vi "Neopixel-Example Dialog.vi"(0 "Cluster In":cluster{"Numeric":dbl}, 2 "Parent VI":refnum<vi>) -> (4 "Cluster out":cluster{"Numeric":dbl}, 10 "canceled":bool)   [LabVIEW 2020]
panel:
  in  "Cancel":bool
  in  "OK":bool
  # "Put stuff here"
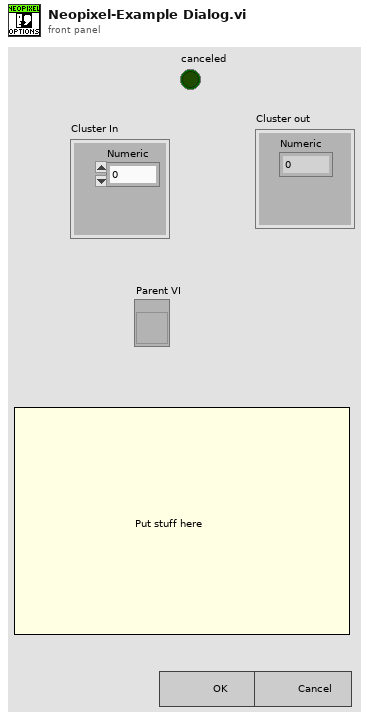
[diagram p1: front panel]
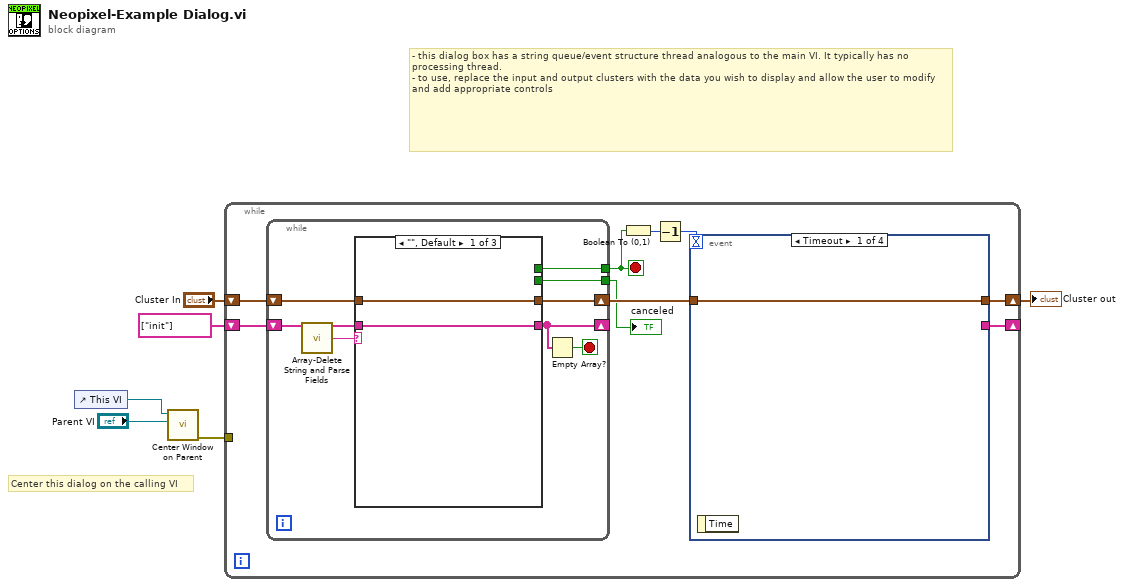
[diagram p0: block diagram]
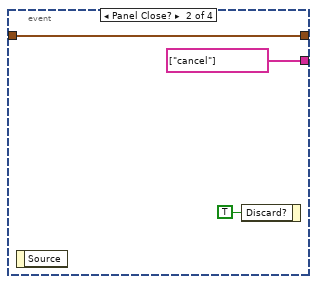
[diagram p2: hidden frame]
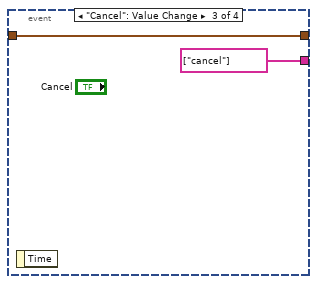
[diagram p3: hidden frame]
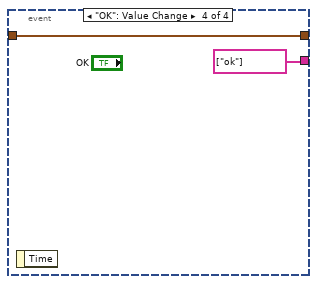
[diagram p4: hidden frame]
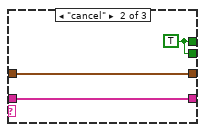
[diagram p5: hidden frame]
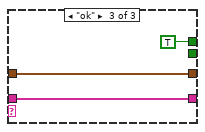
[diagram p6: hidden frame]
diagram:
  # "Center this dialog on the calling VI"
  # "- this dialog box has a string queue/event structure thread analogous to the main VI. It typically has no processing thread.\n- to use, replace the input and output clusters with the data you wish to display and allow the user to modify and add appropriate controls"
  n1 = control-ref of="This VI"() -> (w1:refnum<vi>)
  n2 = call "Center Window on Parent.vi"("Parent VI"="Parent VI", "VI in"=w1) -> ("error out"=w3:errorcluster)  [unwired: 8 in, 1 out]
  n3 = while {
    shift-right: [w9] -> w5
    shift-left: "Cluster In" -> [w15]
    shift-right: [w8] -> _
    shift-left: string[] ["init"] -> [w10]
    tunnel: w3 -> [_]
    stop <- w13 stop-if-true
    n4 = while {
      shift-right: [w31] -> _
      shift-left: w10 -> [w25]
      shift-right: [w28] -> w14
      shift-left: w15 -> [w29]
      tunnel: [w27] -> w13
      tunnel: [w24] -> w7
      stop <- w30 stop-if-true
      n5 = call "Array-Delete String and Parse Fields.vi"("Array in"=w25) -> ("Array out"=w32:string[], "Field 1"=w26:string)  [unwired: 10 in, 3 out]
      n6 = case shown="\"\", Default" w26 {
        tunnel: w32 -> [w34 w37 w40]
        tunnel: [w34 w37 w40] -> w31
        tunnel: w29 -> [w33 w36 w39]
        tunnel: [w33 w36 w39] -> w28
        tunnel: [_ w35 TRUE] -> w27
        tunnel: [_ w35 _] -> w24
        frame "", Default {
        }
        frame "cancel" {
          w35 = TRUE
        }
        frame "ok" {
        }
      }
      n7 = Empty Array?(array=w31) -> (empty?=w30:bool)
    }
    "canceled" <- w7
    n8 = Boolean To (0,1)(Boolean=w13) -> (0, 1=w12:i16)
    n9 = Decrement(x=w12) -> (x-1=w11:i16)
    n10 = event shown="[0] Timeout" {
      selector: _ -> [_ _ _ _]
      dyn-events: _ -> [_ _ _ _]
      timeout: w11 -> [_ _ _ _]
      tunnel: w14 -> [w16 w19 w20 w23]
      tunnel: [w16 w19 w20 w23] -> w9
      tunnel: [_ string[] ["cancel"] string[] ["cancel"] string[] ["ok"]] -> w8
      event Timeout {
        n11 = event-data() -> ()  [unwired: 1 in, 1 out]
      }
      event Panel Close? {
        n12 = event-data() -> ()  [unwired: 1 in, 1 out]
        n13 = event-data("Discard?"=TRUE) -> ()  [unwired: 1 in, 1 out]
      }
      event "Cancel": Value Change {
        n14 = event-data() -> ()  [unwired: 1 in, 1 out]
      }
      event "OK": Value Change {
        n15 = event-data() -> ()  [unwired: 1 in, 1 out]
      }
    }
  }
  "Cluster out" <- w5
